vi "FTW-Package-Multipart-Interpret.vi"(0 "FTW-Message-Lossy In":refnum<class "FTW-Package-Lossy.lvclass">, 11 "error in":errorcluster) -> (4 "FTW-Message-Lossy Out":refnum<class "FTW-Package-Lossy.lvclass">, 6 "Message":T1, 15 "error out":errorcluster)   [LabVIEW 2013, in "FTW-Package-Lossy.lvclass"]
uses:
  FTW-Package-Lossy.lvclass
  Message/FTW-Message.ctl
  FTW-Package-Lossy.lvclass/FTW-Package-Lossy.ctl
panel:
  # "Inputs"
  # "Outputs"
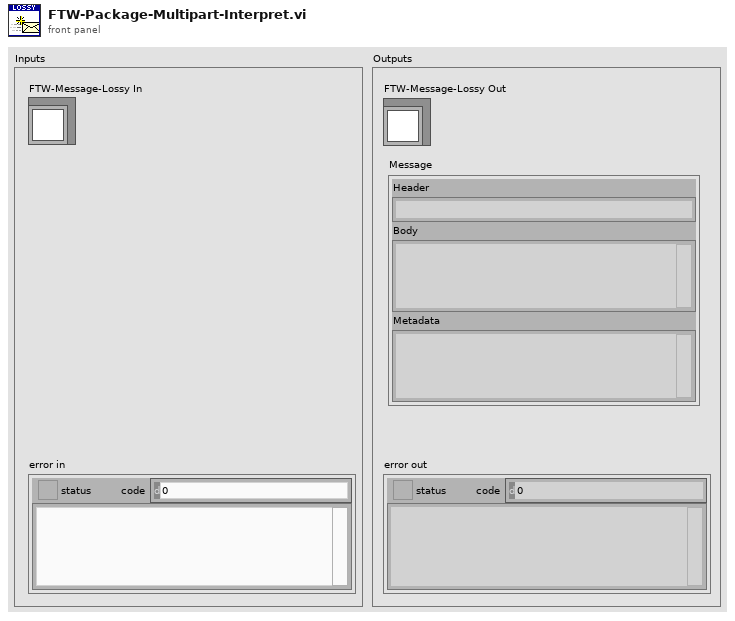
[diagram p1: front panel]
types:
  T1 = typedef "FTW-Message.ctl" = cluster{"Header":string, "Body":string, "Metadata":string}
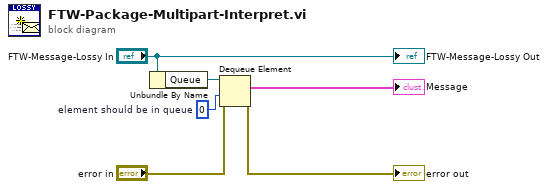
[diagram p0: block diagram]
diagram:
  w2 = 0  # element should be in queue
  n1 = Unbundle By Name("FTW-Message-Lossy In") -> ("Queue"=w5:refnum<queue>)
  n2 = Dequeue Element(queue=w5, timeout in ms (-1)=w2, error in (no error)="error in") -> (element=→"Message":T1, error out=→"error out":errorcluster)  [unwired: 2 out]
  "FTW-Message-Lossy Out" <- "FTW-Message-Lossy In"
